vi "Edges and center.vi"(11 "Class Result":T1 {"Bounding Box"."y" format="%.2f"; "Bounding Box"."x" format="%.2f"}) -> (0 "y2":sgl, 1 "y":sgl, 2 "x2":sgl, 3 "x":sgl, 5 "y center":sgl, 7 "x center":sgl)   [LabVIEW 2020]
uses:
  <vilib>/vision/Deep Learning.llb/IMAQ DL Model Objects.ctl
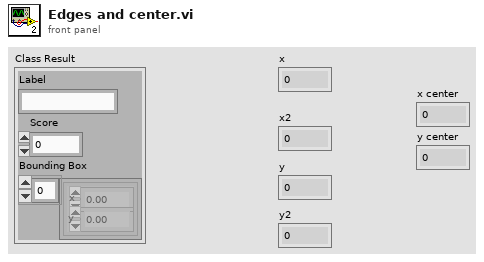
[diagram p1: front panel]
types:
  T1 = typedef "IMAQ DL Model Objects.ctl" = cluster{"Label":string, "Score":sgl, "Bounding Box":cluster{"x":sgl, "y":sgl}[]}
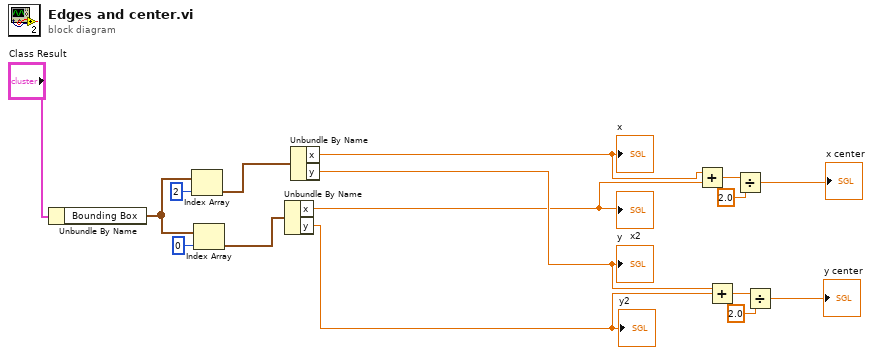
[diagram p0: block diagram]
diagram:
  n1 = Unbundle By Name("Class Result") -> ("Bounding Box"=w13:cluster{"x":sgl, "y":sgl}[])
  n2 = Index Array(array=w13, index=2) -> (element=w12:cluster{"x":sgl, "y":sgl})
  n3 = Index Array(array=w13, index=0) -> (element=w11:cluster{"x":sgl, "y":sgl})
  n4 = Unbundle By Name(w11) -> ("x"=w3:sgl, "y"=w6:sgl)
  "y2" <- w6
  "x2" <- w3
  n5 = Unbundle By Name(w12) -> ("x"=w2:sgl, "y"=w7:sgl)
  "y" <- w7
  "x" <- w2
  n6 = Add(x=w2, y=w3) -> (x+y=w5:sgl)
  n7 = Add(x=w7, y=w6) -> (x+y=w10:sgl)
  n8 = Divide(x=w5, y=sgl 2.0) -> (x/y=→"x center":sgl)
  n9 = Divide(x=w10, y=sgl 2.0) -> (x/y=→"y center":sgl)
